vi "Set timeline cursor color.vi"(9 "Color for Cursor 1":u32, 10 "Color for Cursor 0":u32, 11 "Timeline Graph in":T1) -> (3 "Timeline Graph out":T1)   [LabVIEW 2017, in "XGrapher.xctl"]
uses:
  XGrapher.xctl
  Typedefs/Xctrl-Timeline graph ref.ctl
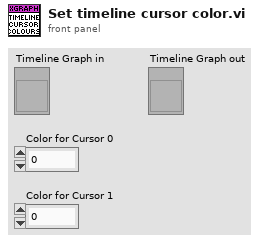
[diagram p1: front panel]
types:
  T1 = typedef "XGrapher.xctl/Xctrl-Timeline graph ref.ctl" = refnum<vi>
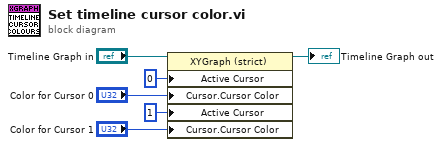
[diagram p0: block diagram]
diagram:
  n1 = property on="Property Node" class="XYGraph (strict)"(reference="Timeline Graph in", "Active Cursor"=u32 0, "Cursor.Cursor Color"="Color for Cursor 0", "Active Cursor"=u32 1, "Cursor.Cursor Color"="Color for Cursor 1") -> (reference out=→"Timeline Graph out":T1)  [unwired: 1 in, 1 out]
